vi "Format Signal Name.vi"(8 "error in (no error)":errorcluster, 11 "String":string) -> (0 "error out":errorcluster, 3 "String out":string)   [LabVIEW 2015, in "Project.lvclass"]
uses:
  Project.lvclass
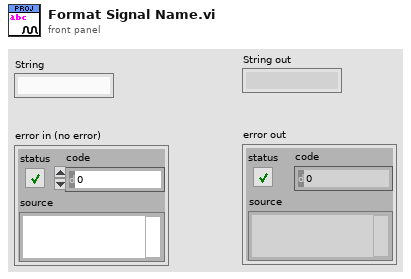
[diagram p1: front panel]
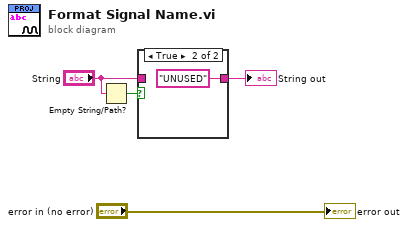
[diagram p0: block diagram]
diagram:
  n1 = Empty String/Path?(string/path="String") -> (empty?=w4:bool)
  n2 = case shown="True" w4 {
    tunnel: "String" -> [w5 _]
    tunnel: [w5 "UNUSED" ("String")] -> w2
    frame False {
    }
    frame True {
    }
  }
  "String out" <- w2
  "error out" <- "error in (no error)"
